vi "Meadowlark Serial IO Example.VI"() -> ()   [LabVIEW 2009]
doc: "This example selects channels and sets and reads voltages on a Meadowlark Optics D3040 Four-Cell controller. This VI can be opened and examined using LabVIEW (6.1 or newer) as a starting point for a user's custom development of a D3040 interface. Please note that the Sub-VI's used in this program require the file \"usbdrvd.dll\".\n\n(c) 2003-2004 Meadowlark Optics, Inc. All rights reserved."
panel:
  out "FW Version":dbl format="%.2f"
  out "Update \nChannel":bool[](array[boolean])
  out "Readout \nVoltages":dbl[](array[numeric]) format="%.3f"
  in  "stop":bool
  in  "VISA \nResource Name":refnum<visa-resource-name>="ASRL1::INSTR"
  in  "Channel":i32=1 min=1 max=4 step=1
  in  "Set Voltage":dbl min=0.0 max=10.0 step=0.001 format="%.3f"
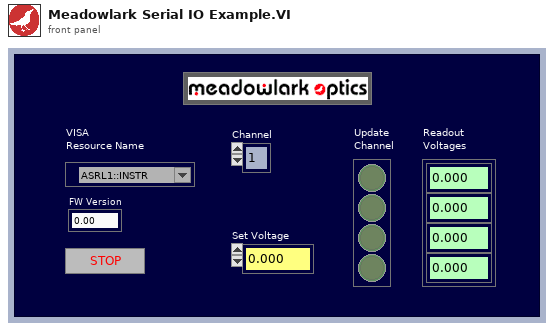
[diagram p1: front panel]
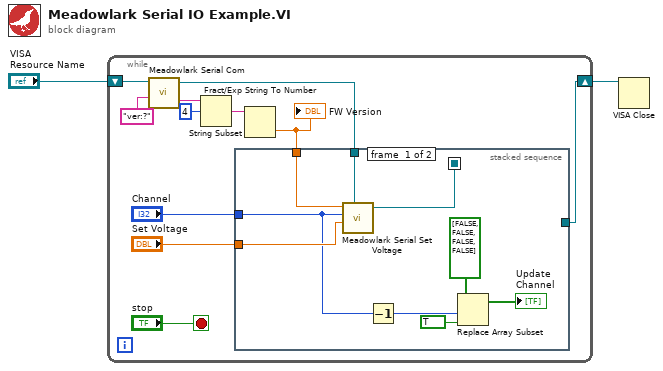
[diagram p0: block diagram]
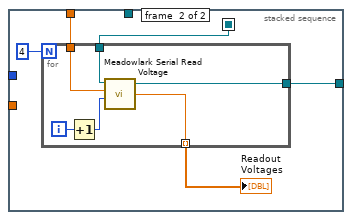
[diagram p2: hidden frame]
diagram:
  n1 = while {
    shift-right: [w10] -> w1
    shift-left: "VISA \nResource Name" -> [w8]
    stop <- "stop" stop-if-true
    n2 = call "Meadowlark Serial Com.VI"("WRITE IN String"="ver:?", "VISA \nResource Name"=w8) -> ("READ OUT String"=w6:string, "Duplicate VISA \nResource Name"=w9:refnum<visa-resource-name>)  [unwired: 2 in, 1 out]
    n3 = String Subset(string=w6, offset (0)=4) -> (substring=w4:string)  [unwired: 1 in]
    n4 = Fract/Exp String To Number(string=w4) -> (number=w3:dbl)  [unwired: 3 in, 1 out]
    "FW Version" <- w3
    n5 = stacked-sequence {
      seq-local: [w16 _] -> [_ w24]
      tunnel: "Set Voltage" -> [w18 _]
      tunnel: "Channel" -> [w17 _]
      tunnel: w9 -> [w15 _]
      tunnel: [_ w25] -> w10
      tunnel: w3 -> [w14 w23]
      frame #0 {
        n6 = call "Meadowlark Serial Set Voltage.VI"("FW Version"=w14, "LC Channel"=w17, "LC Voltage"=w18, "VISA \nResource Name"=w15) -> ("Duplicate VISA \nResource Name"=w16:refnum<visa-resource-name>)  [unwired: 1 in, 2 out]
        n7 = Decrement(x=w17) -> (x-1=w22:i32)
        n8 = Replace Array Subset(array=bool[] [FALSE, FALSE, FALSE, FALSE], new element=TRUE ("new element/subarray"), index=w22) -> (→"Update \nChannel":bool[])
      }
      frame #1 {
        n9 = for {
          N: 4 -> [_]
          tunnel: [w32] -> w26 mode=indexing
          tunnel: w24 -> [w30]
          tunnel: [w29] -> w25
          tunnel: w23 -> [w28]
          i -> [w33]
          n10 = Increment(x=w33) -> (x+1=w31:i32)
          n11 = call "Meadowlark Serial Read Voltage.VI"("LC Channel"=w31, "FW Version"=w28, "VISA \nResource Name"=w30) -> ("Readout \nVoltage"=w32:dbl, "Duplicate VISA \nResource Name"=w29:refnum<visa-resource-name>)  [unwired: 1 in, 1 out]
        }
        "Readout \nVoltages" <- w26
      }
    }
  }
  n12 = VISA Close(VISA resource name=w1) -> ()  [unwired: 1 in, 1 out]
